vi "Read service_name.vi"(8 "error in (no error)":errorcluster, 11 "TCPSettings in":refnum<class "TCPSettings.lvclass">) -> (0 "error out":errorcluster, 2 "service_name":string="tcp", 3 "TCPSettings out":refnum<class "TCPSettings.lvclass">)   [LabVIEW 2016, in "TCPSettings.lvclass"]
uses:
  TCPSettings.lvclass
  TCPSettings.lvclass/TCPSettings.ctl
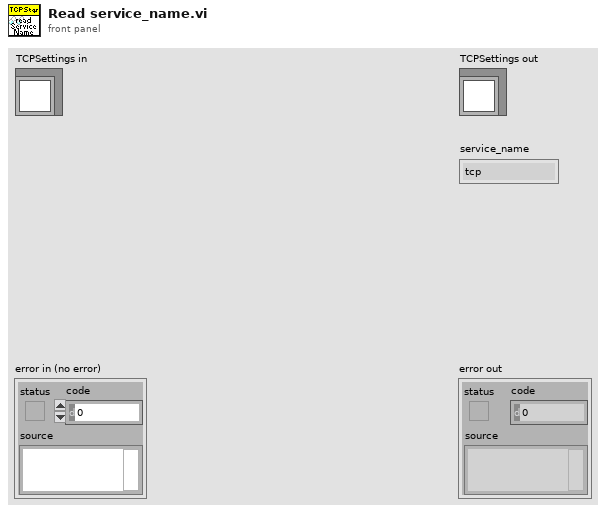
[diagram p1: front panel]
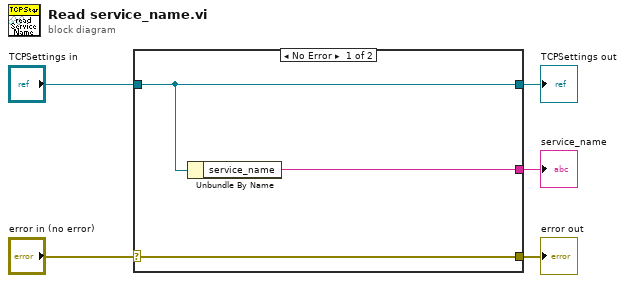
[diagram p0: block diagram]
diagram:
  n1 = case shown="No Error" "error in (no error)" {
    selector: "error in (no error)" -> [w8 w9]
    tunnel: [w8 w9] -> w4
    tunnel: [w7 w10] -> w2
    tunnel: "TCPSettings in" -> [w7 w10]
    tunnel: [w6 _] -> w1
    frame No Error {
      n2 = Unbundle By Name(w7) -> ("service_name"=w6:string)
    }
    frame Error {
    }
  }
  "error out" <- w4
  "TCPSettings out" <- w2
  "service_name" <- w1
